vi "GetObjectData.vi"(8 "ErrorIn":errorcluster, 10 "Object":string, 11 "ReferenceIn":refnum<class "AppConfigJSON.lvclass">) -> (0 "ErrorOut":errorcluster, 1 "Object":T1, 3 "ReferenceOut":refnum<class "AppConfigJSON.lvclass">)   [LabVIEW 2021, in "AppConfigJSON.lvclass"]
uses:
  AppConfigJSON.lvclass
  Interface_TAF_IApplicationConfiguration/IApplicationConfiguration/ObjectDataDetails.ctl
  Interface_TAF_IApplicationConfiguration/IApplicationConfiguration/ObjectData.ctl
  Interface_TAF_IApplicationConfiguration/IApplicationConfiguration/IApplicationConfiguration.lvclass
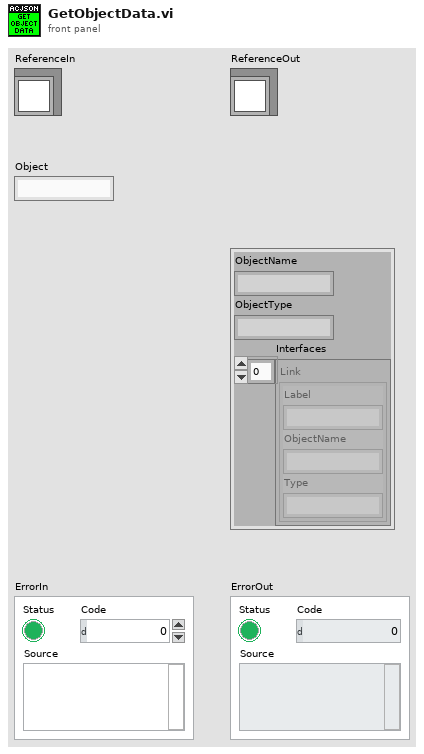
[diagram p1: front panel]
types:
  T1 = typedef "IApplicationConfiguration.lvclass/ObjectDataDetails.ctl" = cluster{"ObjectName":string, "ObjectType":string, "Interfaces":T2[]}
  T2 = typedef "IApplicationConfiguration.lvclass/ObjectData.ctl" = cluster{"Label":string, "ObjectName":string, "Type":string}
  T3 = typedef "AppConfigJSON.lvclass/ObjectAttributes.ctl" = cluster{"Name":string, "ConfigFilePath":path, "Objects":T1[], "ApplicationBasePath":path, "ObjectName":string}
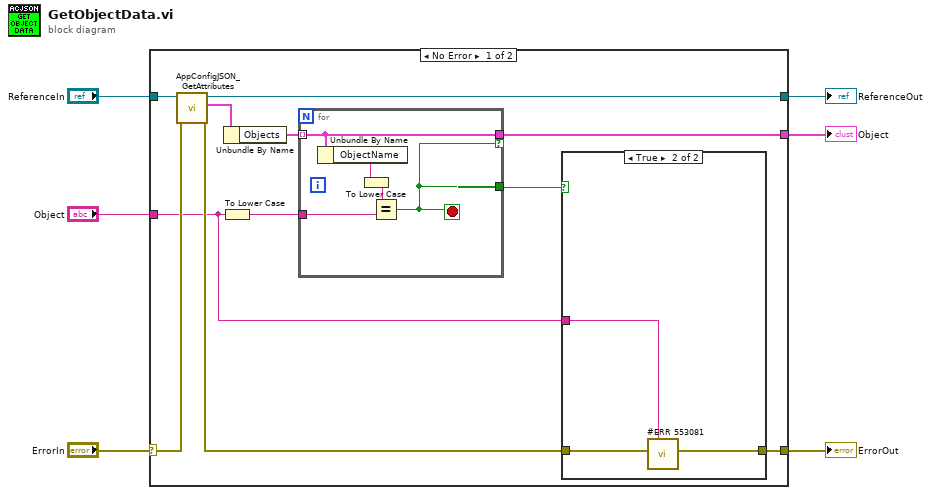
[diagram p0: block diagram]
diagram:
  n1 = case shown="No Error" "ErrorIn" {
    selector: "ErrorIn" -> [w17 w28]
    tunnel: [w16 w28] -> w5
    tunnel: [w12 w27] -> w3
    tunnel: "ReferenceIn" -> [w13 w27]
    tunnel: "Object" -> [w7 _]
    tunnel: [w9 _] -> w1
    frame No Error {
      n2 = call "AppConfigJSON_GetAttributes.vi"("ErrorIn"=w17, "ReferenceIn"=w13) -> ("ErrorOut"=w15:errorcluster, "Data"=w14:T3, "ReferenceOut"=w12:refnum<class "AppConfigJSON.lvclass">)  [unwired: 6 in, 1 out]
      n3 = To Lower Case(string=w7) -> (all lower case string=w10:string)
      n4 = Unbundle By Name(w14) -> ("Objects"=w11:T1[])
      n5 = for {
        tunnel: w10 -> [w26]
        tunnel: w11 -> [w22] mode=indexing
        tunnel: [w22] -> w9 if=w23
        tunnel: [w23] -> w8
        stop <- w23 stop-if-true
        n6 = Unbundle By Name(w22) -> ("ObjectName"=w25:string)
        n7 = To Lower Case(string=w25) -> (all lower case string=w24:string)
        n8 = Equal?(x=w24, y=w26) -> (x = y?=w23:bool)
      }
      n9 = case shown="True" w8 {
        tunnel: w15 -> [w18 w21]
        tunnel: [w18 w20] -> w16
        tunnel: w7 -> [_ w19]
        frame False {
        }
        frame True {
          n10 = call "#ERR 553081"("Data"=w19, "error in (no error)"=w21) -> ("error out"=w20:errorcluster)  [unwired: 9 in]
        }
      }
    }
    frame Error {
    }
  }
  "ErrorOut" <- w5
  "ReferenceOut" <- w3
  "Object" <- w1
